vi "fpga_Position interpolation.vi"(0 "Crossing[U64.16]":fxp<+,64,16> format="%.53g", 1 "Interpolation factor":u16=64, 5 "Stepsize[U64.8]":fxp<+,64,8>, 9 "input valid":bool, 12 "ready for output":bool) -> (4 "resample position [U64.16]":fxp<+,64,16> format="%.53g", 6 "stepsize [U64.8]":fxp<+,64,8>, 10 "output valid":bool, 14 "ready for input":bool)   [LabVIEW 2011, in "NI_EP_Resample_FPGA.lvlib"]
uses:
  <vilib>/addons/Electrical Power/PQ/Resampling/NI_EP_Resample_FPGA.lvlib
  <vilib>/rvi/FXPMathLib/FxpAdd/XNode/nifxpmath_Add.xnode
  <vilib>/rvi/FXPMathLib/basic elements/FxpDiscreteDelay/XNode/nifxpmath_DiscreteDelay.xnode
  <vilib>/rvi/FXPMathLib/sim/FxpSim.dll
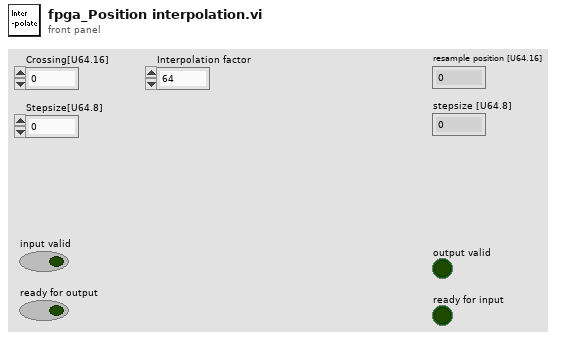
[diagram p1: front panel]
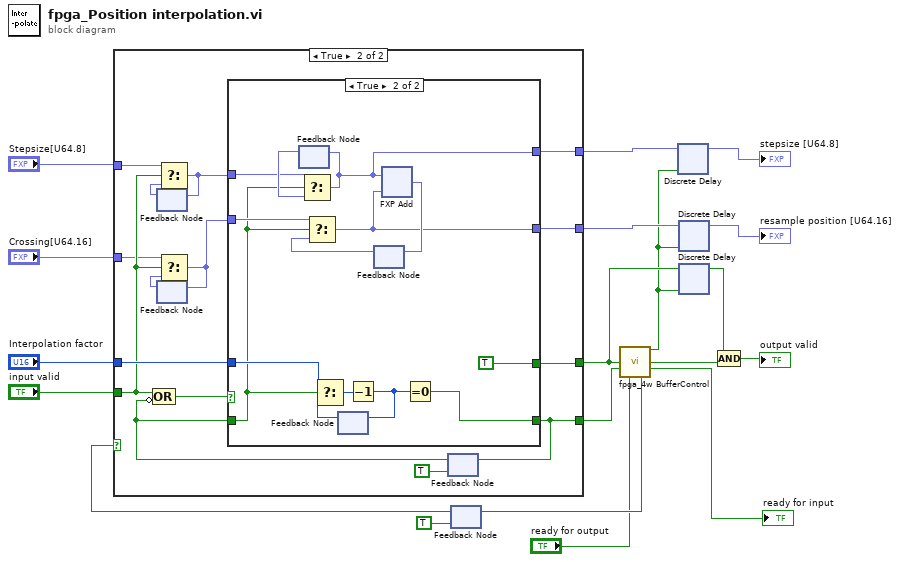
[diagram p0: block diagram]
diagram:
  n1 = feedback #1(TRUE ("logic enable")) -> (w12:bool)
  n2 = case shown="True" w12 {
    tunnel: "Interpolation factor" -> [_ w34]
    tunnel: "Crossing[U64.16]" -> [_ w21]
    tunnel: "input valid" -> [_ w22]
    tunnel: [_ w33] -> w15
    tunnel: [_ w32] -> w11
    tunnel: "Stepsize[U64.8]" -> [_ w26]
    tunnel: [_ w31] -> w14
    tunnel: [_ w27] -> w5
    frame False {
    }
    frame True {
      n3 = feedback #2() -> (w25:fxp<+,64,8>)  [unwired: 1 in]
      n4 = feedback #3() -> (w23:fxp<+,64,16>)  [unwired: 1 in]
      n5 = Select(t=w26, s=w22, f=w25) -> (s? t:f=w24:fxp<+,64,8>)
      n6 = feedback-in #2(w24) -> ()
      n7 = Select(t=w21, s=w22, f=w23) -> (s? t:f=w20:fxp<+,64,16>)
      n8 = feedback-in #3(w20) -> ()
      n9 = feedback #4(TRUE) -> (w28:bool)
      n10 = Compound Arithmetic op=OR(w22, invert w28) -> (w29:bool)
      n11 = case shown="True" w29 {
        tunnel: w34 -> [_ w49]
        tunnel: w20 -> [_ w39]
        tunnel: [_ w46] -> w33
        tunnel: [_ TRUE] -> w32
        tunnel: [w35 w42] -> w31
        tunnel: w24 -> [_ w41]
        tunnel: w28 -> [w35 w37]
        tunnel: [_ w40] -> w27
        frame False {
        }
        frame True {
          n12 = feedback #5() -> (w44:fxp<+,64,8>)  [unwired: 1 out]
          n13 = Select(t=w41, s=w37, f=w44) -> (s? t:f=w40:fxp<+,64,8>)
          n14 = feedback-in #5(w40) -> ()
          n15 = feedback #6() -> (w48:u16)  [unwired: 1 out]
          n16 = Select(t=w49, s=w37, f=w48) -> (s? t:f=w45:u16)
          n17 = Decrement(x=w45) -> (x-1=w43:u16)
          n18 = feedback-in #6(w43) -> ()
          n19 = feedback #7() -> (w38:fxp<+,64,16>)  [unwired: 1 out]
          n20 = Select(t=w39, s=w37, f=w38) -> (s? t:f=w46:fxp<+,64,16>)
          n21 = xnode "FXP Add"("x"=w40, "y"=w46) -> ("x+y"=w47:fxp<+,64,16>)
          n22 = feedback-in #7(w47) -> ()
          n23 = Equal To 0?(x=w43) -> (x = 0?=w42:bool)
        }
      }
      n24 = feedback-in #4(w31) -> ()
    }
  }
  n25 = call <vilib>:"fpga_4w BufferControl.vi"("DR"=w11, "RFI"=w14, "RFO"="ready for output") -> ("buff enable"=w4:bool, "output valid"=w2:bool, "ready for input"=→"ready for input":bool, "logic enable"=w17:bool)  [unwired: 9 in]
  n26 = feedback-in #1(w17) -> ()
  n27 = xnode "Discrete Delay"("D"=w5, "enable"=w4) -> ("Q"=→"stepsize [U64.8]":fxp<+,64,8>)
  n28 = xnode "Discrete Delay"("D"=w15, "enable"=w4) -> ("Q"=→"resample position [U64.16]":fxp<+,64,16>)
  n29 = xnode "Discrete Delay"("D"=w11, "enable"=w4) -> ("Q"=w10:bool)
  n30 = Compound Arithmetic op=AND(w10, w2) -> (→"output valid":bool)
